vi "format_configuration_parameterless_commands.vi"(8 "error in (no error)":errorcluster, 10 "Configuration editables":T1(array[cluster])=[{"INI key name"="FieldCurrentRatio", "Configuration command"="CONF:COIL"}, {"INI key name"="HasPSwitch", "Configuration command"="CONF:PS"}, {"INI key name"="SwitchHtrCurrent", "Configuration command"="CONF:PS:CURR"}, {"INI key name"="SwitchWaitTime", "Configuration command"="CONF:PS:HTIME"}, {"INI key name"="SwitchWaitTime", "Configuration command"="CONF:PS:CTIME"}, {"INI key name"="SwitchCoolingGain", "Configuration command"="CONF:PS:CGAIN"}, {"INI key name"="StabilitySetting", "Configuration command"="CONF:STAB"}, {"INI key name"="MaxCurrent", "Configuration command"="CONF:CURR:RATING"}, {"INI key name"="MaxCurrent", "Configuration command"="CONF:CURR:LIM"}, {"INI key name"="LimitCurrent", "Configuration command"="CONF:CURR:LIM"}, {"INI key name"="QuenchDetectEnable", "Configuration command"="CONF:QU:DET"}, {"INI key name"="QuenchDetectRate", "Configuration command"="CONF:QU:RATE"}, {"INI key name"="AbsorberPresent", "Configuration command"="CONF:AB"}, {"INI key name"="SwitchPSRampRate", "Configuration command"="CONF:PS:PSRR"}], 11 "Config data in":variant) -> (0 "error out":errorcluster, 3 "Configuration commands":string[](array[string]))   [LabVIEW 2021]
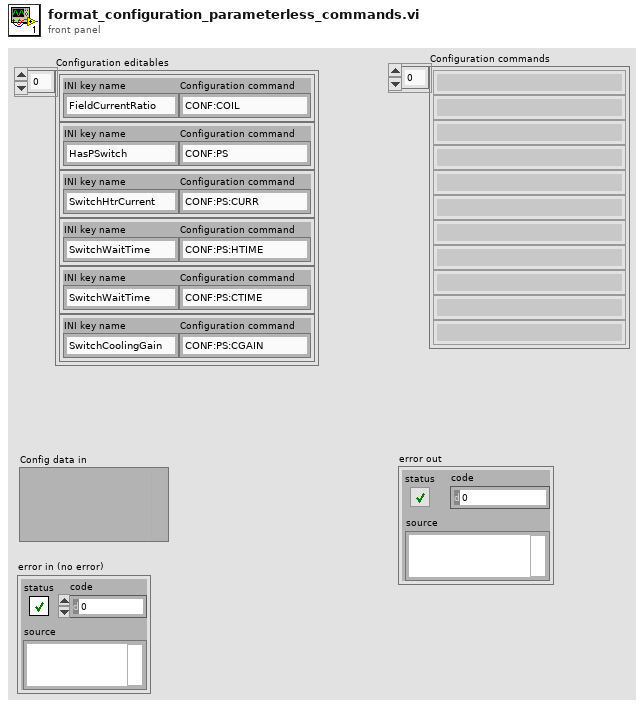
[diagram p1: front panel]
types:
  T1 = cluster{"INI key name":string, "Configuration command":string}[]
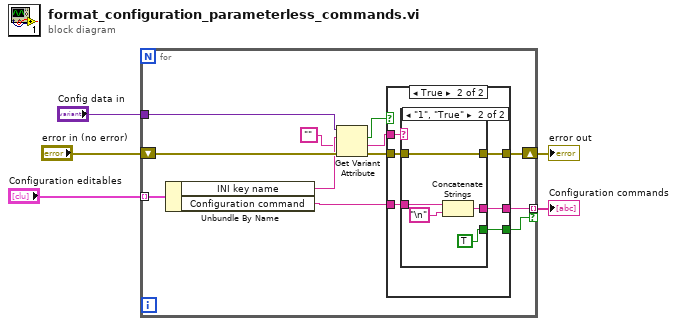
[diagram p0: block diagram]
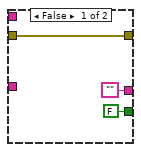
[diagram p2: hidden frame]
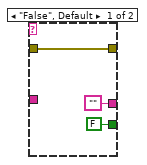
[diagram p3: hidden frame]
diagram:
  n1 = for {
    tunnel: "Configuration editables" -> [w15] mode=indexing
    tunnel: "Config data in" -> [w17]
    shift-right: [w8] -> w2
    shift-left: "error in (no error)" -> [w16]
    tunnel: [w7] -> w1 mode=indexing if=w6
    n2 = Unbundle By Name(w15) -> ("INI key name"=w14:string, "Configuration command"=w11:string)
    n3 = Get Variant Attribute(Variant=w17, name=w14, default value (empty Variant)="", error in=w16) -> (found=w12:bool, value=w10:string, error out=w9:errorcluster)  [unwired: 1 out]
    n4 = case shown="True" w12 {
      tunnel: w11 -> [_ w22]
      tunnel: w10 -> [_ w24]
      tunnel: ["" w21] -> w7
      tunnel: w9 -> [w20 w26]
      tunnel: [w20 w25] -> w8
      tunnel: [FALSE w23] -> w6
      frame False {
      }
      frame True {
        n5 = case shown="\"1\", \"True\"" w24 {
          tunnel: w26 -> [w29 w34]
          tunnel: [w29 w34] -> w25
          tunnel: ["" w30] -> w21
          tunnel: [FALSE TRUE] -> w23
          tunnel: w22 -> [_ w32]
          frame "False", Default {
          }
          frame "1", "True" {
            n6 = Concatenate Strings(w32, "\n") -> (w30:string)
          }
        }
      }
    }
  }
  "Configuration commands" <- w1
  "error out" <- w2
